vi "Rational Interpolation PtByPt.vi"(0 "y":dbl format="%0.2f", 1 "x":dbl format="%0.2f", 2 "sample length":i32=10, 3 "x value":dbl format="%0.2f", 4 "initialize":bool) -> (5 "interpolation value":dbl format="%0.2f", 6 "interpolation error":dbl format="%0.2f", 7 "error":i32)   [LabVIEW 2017, in "NI_PtbyPt.lvlib"]
doc: "Interpolates or extrapolates the function f at <B>x</B> using a rational function."
uses:
  <vilib>/ptbypt/NI_PtbyPt.lvlib
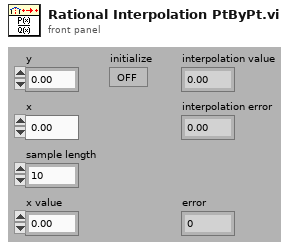
[diagram p1: front panel]
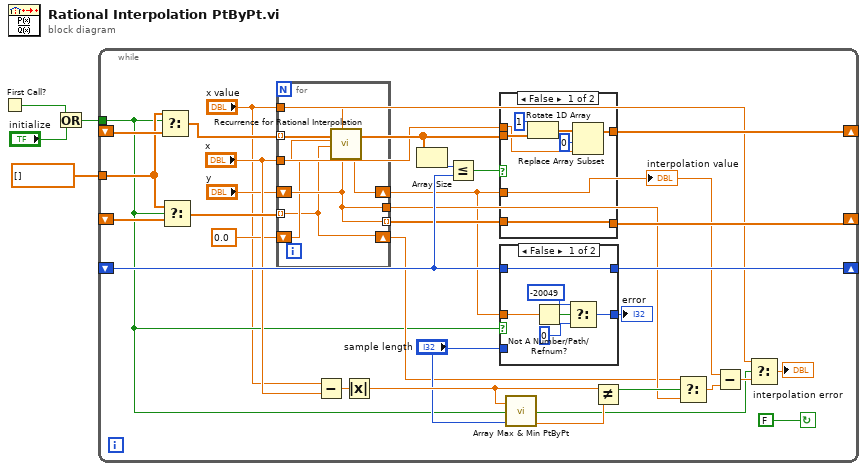
[diagram p0: block diagram]
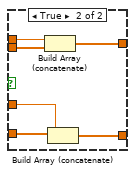
[diagram p2: hidden frame]
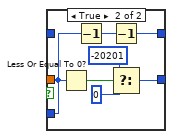
[diagram p3: hidden frame]
diagram:
  n1 = First Call?() -> (First Call?: T/F=w4:bool)
  n2 = Or(x=w4, y="initialize") -> (x .or. y?=w2:bool)
  n3 = while {
    shift-left: _ -> [w26]
    shift-right: [w27] -> _
    tunnel: dbl[] [] ("t") -> [w31]
    tunnel: w2 -> [w7]
    shift-left: _ -> [w33]
    shift-right: [w21] -> _
    shift-left: _ -> [w32]
    shift-right: [w34] -> _
    stop <- FALSE continue-if-true
    n4 = Select(t=w31, s=w7, f=w32) -> (s? t:f=w29:dbl[])
    n5 = Select(t=w31, s=w7, f=w33) -> (s? t:f=w24:dbl[])
    n6 = for {
      shift-right: [w64] -> w11
      shift-left: "y" -> [w63]
      tunnel: w29 -> [w67] mode=indexing
      tunnel: "x" -> [w66]
      tunnel: w24 -> [w61] mode=indexing
      tunnel: "x value" -> [w65]
      tunnel: [w63] -> w22 mode=indexing
      tunnel: [w63] -> w12
      shift-right: [w61] -> w9
      shift-left: 0.0 ("input data x") -> [w62]
      n7 = call <vilib>:"Recurrence for Rational Interpolation.vi"("R(i+1)...(i+m)"=w63, "x"=w65, "R(i+1)...(i+m-1)"=w62, "R(i)...(i+m-1)"=w61, "x2"=w66, "x1"=w67) -> ("Ri(i+1)...(i+m)"=w64:dbl)
    }
    "interpolation value" <- w11
    n8 = Subtract(x="x value", y="x") -> (x-y=w19:dbl)
    n9 = Absolute Value(x=w19) -> (abs(x)=w16:dbl)
    n10 = Array Size(array=w29) -> (size(s)=w28:i32)
    n11 = Less Or Equal?(x=w28, y=w26) -> (x <= y?=w23:bool)
    n12 = case shown="False" w23 {
      tunnel: [w39 w47] -> w34
      tunnel: "x" -> [w36 w46]
      tunnel: w29 -> [w41 w45]
      tunnel: w22 -> [w35 w44]
      tunnel: w11 -> [_ w43]
      tunnel: [w35 w42] -> w21
      frame False {
        n13 = Rotate 1D Array(1:w41, 2:1 ("n")) -> (0:w38:dbl[])
        n14 = Replace Array Subset(array=w38, new element=w36, index=0 ("Index")) -> (w39:dbl[])
      }
      frame True {
        n15 = Build Array (concatenate)(w46, w45) -> (w47:dbl[])
        n16 = Build Array (concatenate)(w44, w43) -> (w42:dbl[])
      }
    }
    n17 = case shown="False" w7 {
      tunnel: "sample length" -> [_ w56]
      tunnel: [w49 w59] -> w30
      tunnel: w11 -> [w53 _]
      tunnel: [w48 w55] -> w27
      tunnel: w26 -> [w48 _]
      frame False {
        n18 = Not A Number/Path/Refnum?(number/path/refnum=w53) -> (NaN/Path/Refnum?=w52:bool)
        n19 = Select(t=-20049, s=w52, f=0) -> (s? t:f=w49:i32)
      }
      frame True {
        n20 = Less Or Equal To 0?(x=w56) -> (x <= 0?=w60:bool)
        n21 = Decrement(x=w56) -> (x-1=w54:i32)
        n22 = Decrement(x=w54) -> (x-1=w55:i32)
        n23 = Select(t=-20201 ("f"), s=w60, f=0 ("t")) -> (s? t:f=w59:i32)
      }
    }
    "error" <- w30
    n24 = call <vilib>:"Array Max & Min PtByPt.vi"("input data point"=w16, "sample length"="sample length", "initialize"=w7) -> ("min value"=w14:dbl)  [unwired: 4 out]
    n25 = Not Equal?(x=w16, y=w14) -> (x != y?=w17:bool)
    n26 = Select(t=w9, s=w17, f=w12) -> (s? t:f=w18:dbl)
    n27 = Subtract(x=w11, y=w18) -> (x-y=w8:dbl)
    n28 = Select(t="x value", s=w7, f=w8) -> (s? t:f=→"interpolation error":dbl)
  }
